vi "Test Leap Years.vi"(8 "error in":errorcluster) -> (0 "error out":errorcluster)   [LabVIEW 2013]
uses:
  source/isLeapYear (integer).vi
  <vilib>/addons/_JKI Toolkits/Caraya/classes/Test/Test.lvclass
  <vilib>/addons/_JKI Toolkits/Caraya/classes/Assert/Assert.lvclass
  <vilib>/addons/_JKI Toolkits/Caraya/classes/Assert/Assert True.vi
  <vilib>/addons/_JKI Toolkits/Caraya/classes/Assert/Assert False.vi
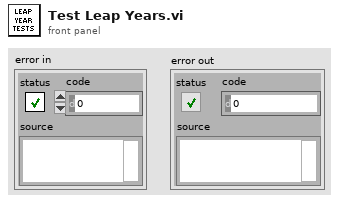
[diagram p1: front panel]
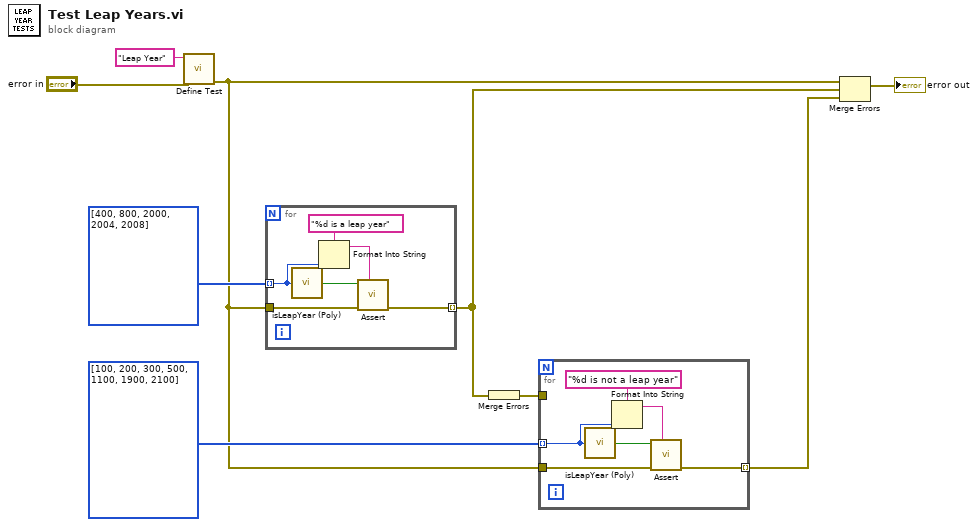
[diagram p0: block diagram]
diagram:
  n1 = call <vilib>:"Define Test.vi"("error in (no error)"="error in", "Label (VI Title)"="Leap Year") -> ("error out"=w1:errorcluster)  [unwired: 8 in, 1 out]
  n2 = for {
    tunnel: i32[] [400, 800, 2000, 2004, 2008] -> [w14] mode=indexing
    tunnel: [w12] -> w3 mode=indexing
    tunnel: w1 -> [w11]
    n3 = call-poly "isLeapYear (Poly).vi"("Year (0: this year)"=w14) -> ("is Leap Year?"=w15:bool)  [unwired: 8 in]
    n4 = Format Into String(format string="%d is a leap year", w14) -> (resulting string=w13:string)  [unwired: 2 in, 1 out]
    n5 = call-poly <vilib>:"Assert.vi"("Label"=w13, "error in (no error)"=w11, "True?"=w15) -> ("error out"=w12:errorcluster)  [unwired: 7 in, 1 out]
  }
  n6 = Merge Errors(w3) -> (w2:errorcluster)
  n7 = for {
    tunnel: i32[] [100, 200, 300, 500, 1100, 1900, 2100] -> [w20] mode=indexing
    tunnel: [w18] -> w4 mode=indexing
    tunnel: w1 -> [w17]
    tunnel: w2 -> [_]
    n8 = call-poly "isLeapYear (Poly).vi"("Year (0: this year)"=w20) -> ("is Leap Year?"=w21:bool)  [unwired: 8 in]
    n9 = Format Into String(format string="%d is not a leap year", w20) -> (resulting string=w19:string)  [unwired: 2 in, 1 out]
    n10 = call-poly <vilib>:"Assert.vi"("Label"=w19, "error in (no error)"=w17, "False?"=w21) -> ("error out"=w18:errorcluster)  [unwired: 7 in, 1 out]
  }
  n11 = Merge Errors(w1, w3, w4) -> (→"error out":errorcluster)
